vi "Config Logging Dialog.vi"(8 "error in (no error)":errorcluster, 10 "New Config (in)":T1={"Log Directory Path"=path "", "Log File Path"=path "", "Log File Prefix"="Experiment", "Log File Extension"="csv", "File Delimiter"=",", "Header Info"=[], "Channels"=[], "Log Instrument Runs"=FALSE}, 11 "Current Config":T1={"Log Directory Path"=path "", "Log File Path"=path "", "Log File Prefix"="Experiment", "Log File Extension"="csv", "File Delimiter"=",", "Header Info"=[], "Channels"=[], "Log Instrument Runs"=FALSE}) -> (0 "error out":errorcluster, 3 "New Config (out)":T1={"Log Directory Path"=path "", "Log File Path"=path "", "Log File Prefix"="Experiment", "Log File Extension"="csv", "File Delimiter"=",", "Header Info"=[], "Channels"=[], "Log Instrument Runs"=FALSE})   [LabVIEW 2020, in "SQSnobFit Control Panel.lvlib" / "Logging.lvlib"]
uses:
  Logging.lvlib
  Logging Configuration.ctl
  Config Logging State.ctl
panel:
  in  "Log Instrument Runs":bool=TRUE
  in  "Experiment Name":string
  in  "File Delimiter":string=","
  in  "Log Directory Path":path
  in  "Save Config Btn":bool
  # "Logging Configuration"
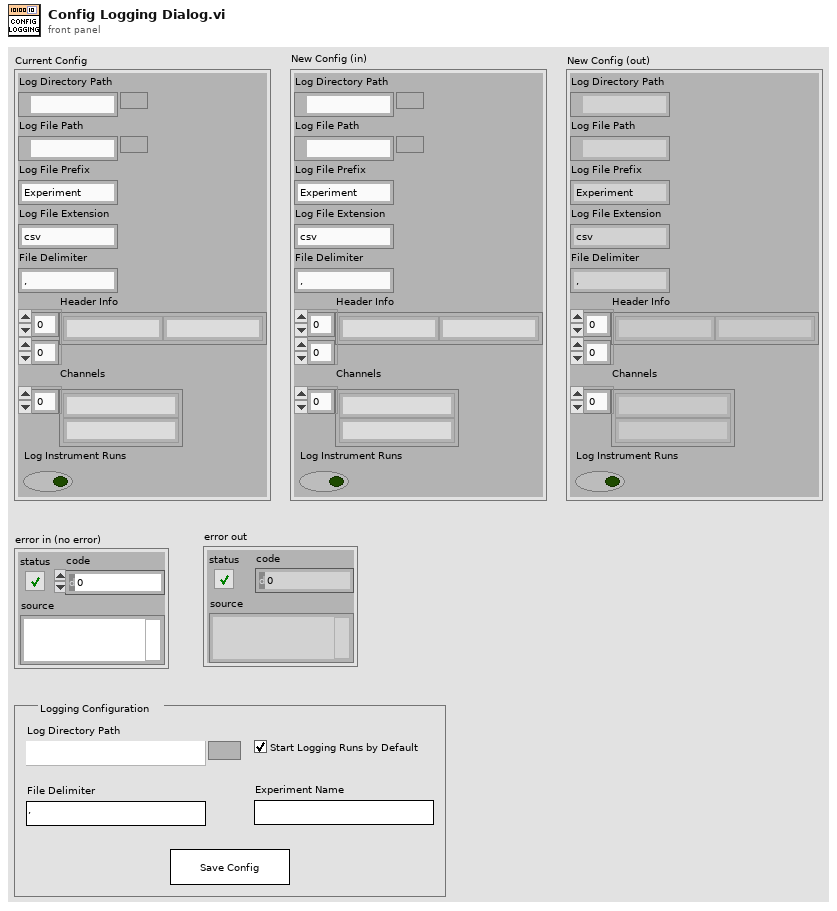
[diagram p1: front panel]
types:
  T1 = typedef "SQSnobFit Control Panel.lvlib/Logging.lvlib/Logging Configuration.ctl" = cluster{"Log Directory Path":path, "Log File Path":path, "Log File Prefix":string, "Log File Extension":string, "File Delimiter":string, "Header Info":string[][], "Channels":string[], "Log Instrument Runs":bool}
  T2 = typedef "SQSnobFit Control Panel.lvlib/Logging.lvlib/Config Logging State.ctl" = enum16{"Initializing", "Waiting for save", "Saving", "Closing"}
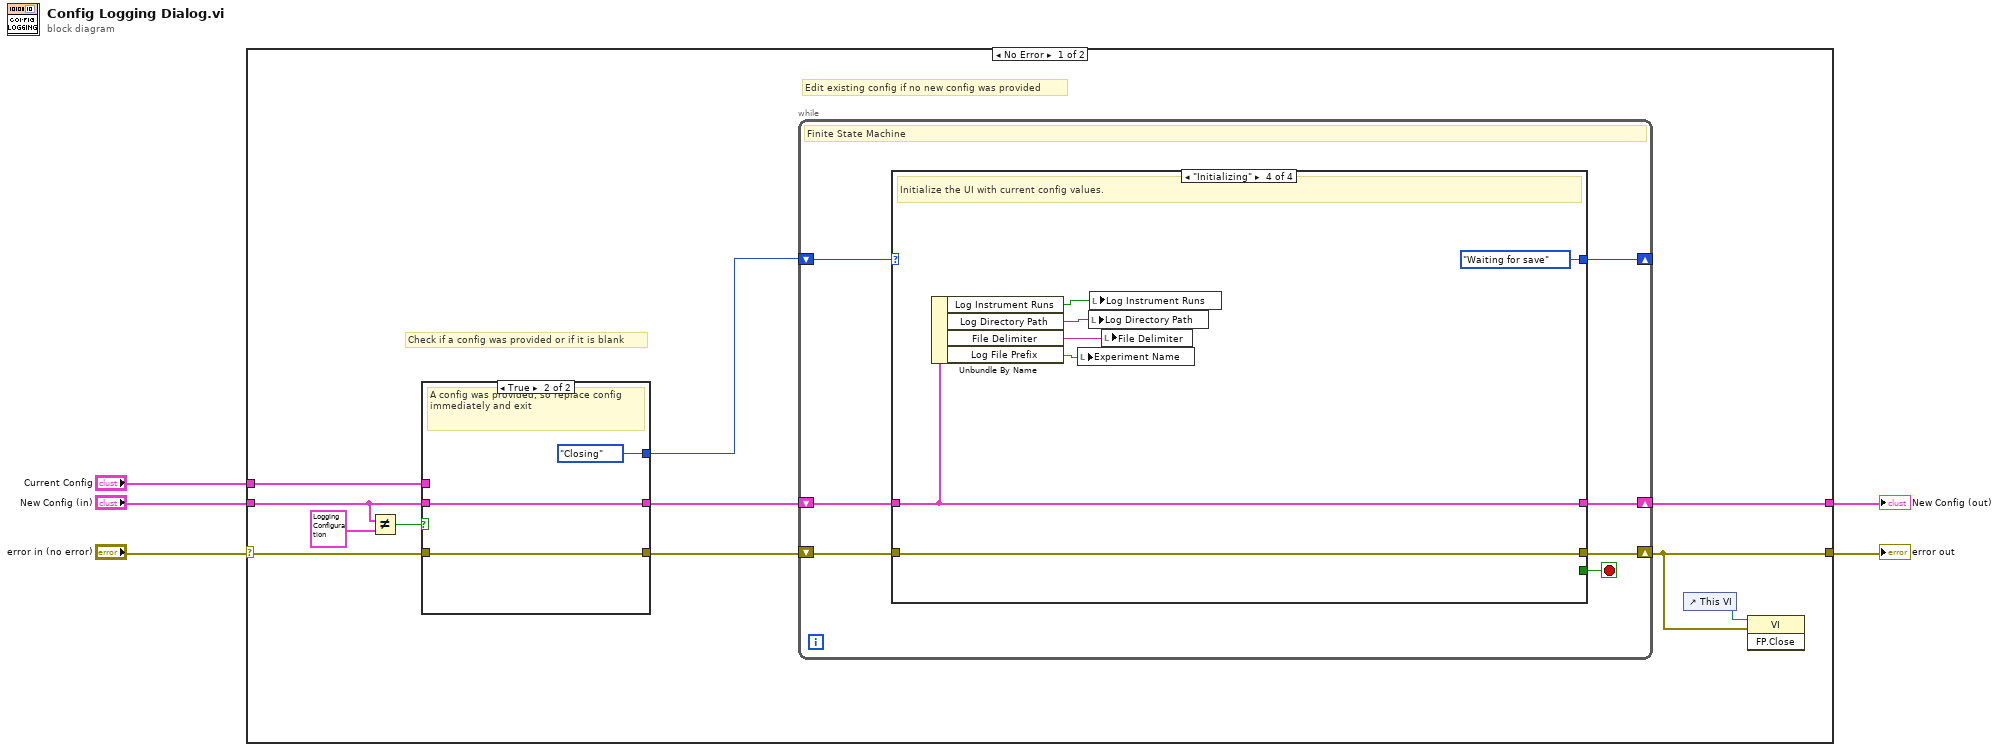
[diagram p0: block diagram]
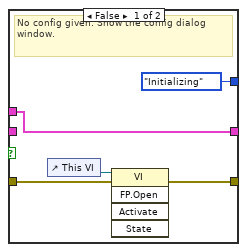
[diagram p2: hidden frame]
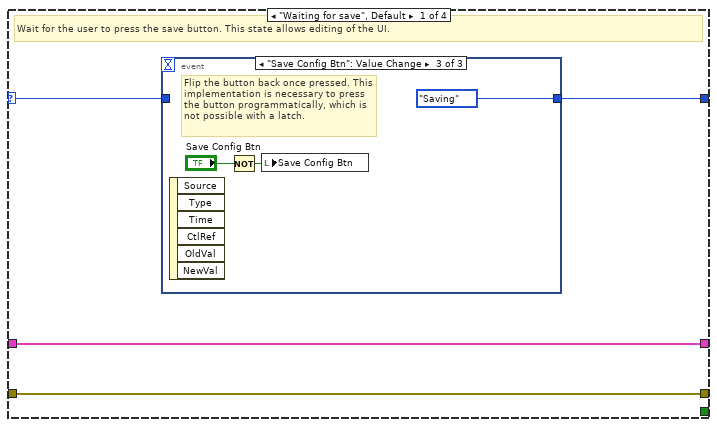
[diagram p3: hidden frame]
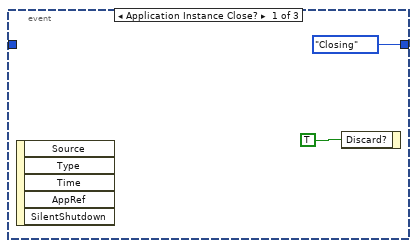
[diagram p4: hidden frame]
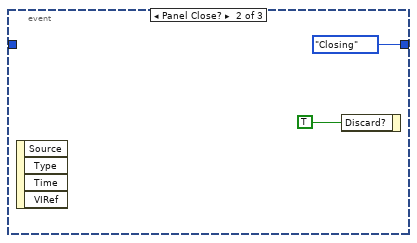
[diagram p5: hidden frame]
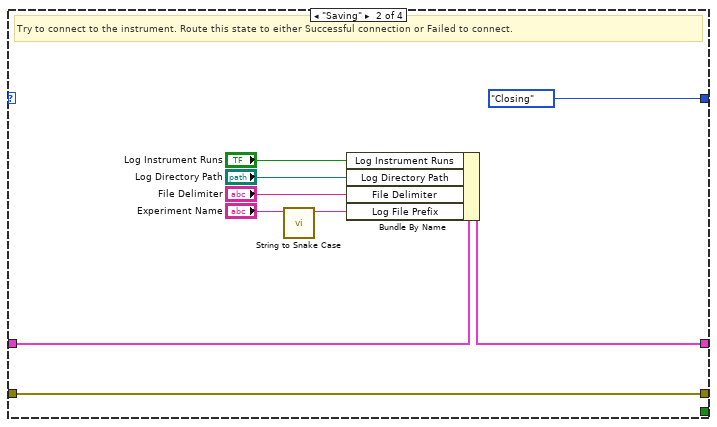
[diagram p6: hidden frame]
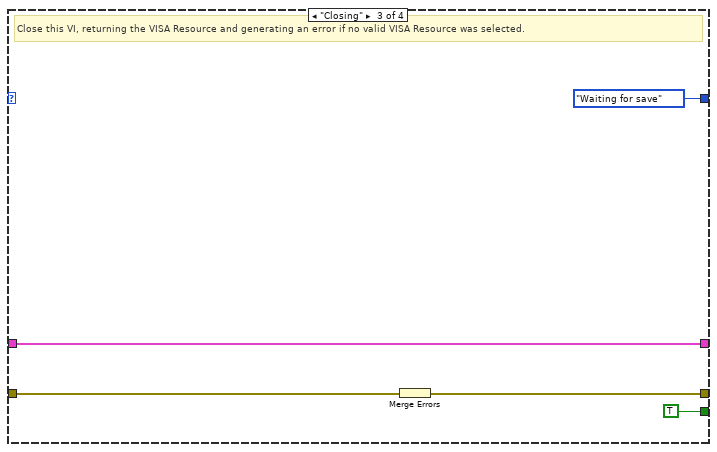
[diagram p7: hidden frame]
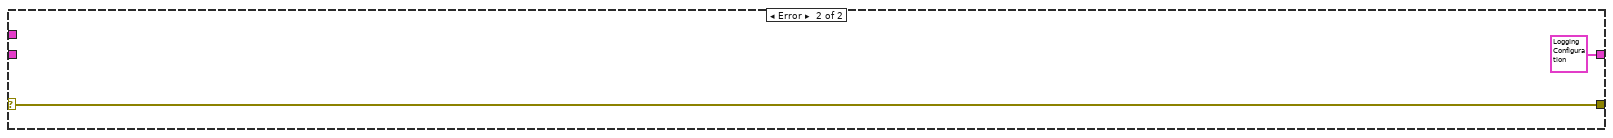
[diagram p8: hidden frame]
diagram:
  n1 = case shown="No Error" "error in (no error)" {
    selector: "error in (no error)" -> [w11 w65]
    tunnel: [w16 T1 {"Log Directory Path"=path "", "Log File Path"=path "", "Log File Prefix"="Experiment", "Log File Extension"="csv", "File Delimiter"=",", "Header Info"=[], "Channels"=[], "Log Instrument Runs"=FALSE} ("New Config (in)")] -> w2
    tunnel: [w14 w65] -> w3
    tunnel: "New Config (in)" -> [w8 _]
    tunnel: "Current Config" -> [w6 _]
    frame No Error {
      # "Edit existing config if no new config was provided"
      # "Check if a config was provided or if it is blank"
      n2 = Not Equal?(x=w8, y=T1 {"Log Directory Path"=path "", "Log File Path"=path "", "Log File Prefix"="Experiment", "Log File Extension"="csv", "File Delimiter"=",", "Header Info"=[], "Channels"=[], "Log Instrument Runs"=FALSE} ("Old Config")) -> (x != y?=w13:bool)
      n3 = case shown="True" w13 {
        tunnel: w11 -> [w20 w24]
        tunnel: [w19 w24] -> w10
        tunnel: [Config_Logging_State."Initializing" Config_Logging_State."Closing"] -> w9
        tunnel: w8 -> [_ w22]
        tunnel: [w17 w22] -> w7
        tunnel: w6 -> [w17 _]
        frame False {
          # "No config given. Show the config dialog window."
          n4 = control-ref of="This VI"() -> (w21:refnum<vi>)
          n5 = invoke class="VI" method="FP.Open"(reference=w21, error in=w20) -> (error out=w19:errorcluster)  [unwired: 3 in, 4 out]
        }
        frame True {
          # "A config was provided, so replace config immediately and exit"
        }
      }
      n6 = while {
        shift-right: [w30] -> _
        shift-left: w9 -> [w31]
        shift-right: [w28] -> w16
        shift-left: w7 -> [w27]
        shift-right: [w25] -> w14
        shift-left: w10 -> [w26]
        stop <- w29 stop-if-true
        # "Finite State Machine"
        n7 = case shown="\"Initializing\"" w31 {
          selector: w31 -> [w35 _ _ _]
          tunnel: [w34 Config_Logging_State."Closing" Config_Logging_State."Waiting for save" Config_Logging_State."Waiting for save"] -> w30
          tunnel: [_ _ TRUE _] -> w29
          tunnel: [w32 w49 w55 w57] -> w28
          tunnel: w27 -> [w32 w43 w55 w57]
          tunnel: w26 -> [w33 w51 w53 w59]
          tunnel: [w33 w51 w54 w59] -> w25
          frame "Waiting for save", Default {
            # "Wait for the user to press the save button. This state allows editing of the UI."
            n8 = event shown="[2] \"Save Config Btn\": Value Change" {
              selector: _ -> [_ _ _]
              dyn-events: _ -> [_ _ _]
              timeout: _ -> [_ _ _]
              tunnel: [Config_Logging_State."Closing" Config_Logging_State."Closing" Config_Logging_State."Saving"] -> w34
              tunnel: w35 -> [_ _ _]
              event Application Instance Close? {
                n9 = event-data() -> ()  [unwired: 1 in, 5 out]
                n10 = event-data("Discard?"=TRUE) -> ()  [unwired: 1 in, 1 out]
              }
              event Panel Close? {
                n11 = event-data() -> ()  [unwired: 1 in, 4 out]
                n12 = event-data("Discard?"=TRUE) -> ()  [unwired: 1 in, 1 out]
              }
              event "Save Config Btn": Value Change {
                # "Flip the button back once pressed. This implementation is necessary to press the button programmatically, which is not possible with a latch."
                n13 = event-data() -> ()  [unwired: 1 in, 6 out]
                n14 = Not(x="Save Config Btn") -> (.not. x?=w41:bool)
                n15 = local write "Save Config Btn"(w41) -> ()
              }
            }
          }
          frame "Saving" {
            # "Try to connect to the instrument. Route this state to either Successful connection or Failed to connect."
            n16 = call "String to Snake Case.vi"("String"="Experiment Name") -> ("Snake Case String"=w45:string)  [unwired: 10 in]
            n17 = Bundle By Name(cluster=w43, "Log Instrument Runs"="Log Instrument Runs", "Log Directory Path"="Log Directory Path", "File Delimiter"="File Delimiter", "Log File Prefix"=w45) -> (w49:T1)
          }
          frame "Closing" {
            # "Close this VI, returning the VISA Resource and generating an error if no valid VISA Resource was selected."
            n18 = Merge Errors(w53) -> (w54:errorcluster)
          }
          frame "Initializing" {
            # "Initialize the UI with current config values."
            n19 = Unbundle By Name(w57) -> ("Log Instrument Runs"=w58:bool, "Log Directory Path"=w63:path, "File Delimiter"=w62:string, "Log File Prefix"=w61:string)
            n20 = local write "Experiment Name"(w61) -> ()
            n21 = local write "Log Directory Path"(w63) -> ()
            n22 = local write "Log Instrument Runs"(w58) -> ()
            n23 = local write "File Delimiter"(w62) -> ()
          }
        }
      }
      n24 = control-ref of="This VI"() -> (w15:refnum<vi>)
      n25 = invoke class="VI" method="FP.Close"(reference=w15, error in=w14) -> ()  [unwired: 1 in, 3 out]
    }
    frame Error {
    }
  }
  "New Config (out)" <- w2
  "error out" <- w3
